vi "svx_Oct_Autoscale Ranges.vi"(10 "Display State In":T1={"X Scale Width %"=50.0, "Y Scale Height %"=50.0, "X-Axis Range"={"Minimum"=0.0, "Maximum"=10.0}, "Y-Axis Range"={"Minimum"=0.0, "Maximum"=10.0}, "Z-Axis Range"={"Minimum"=0.0, "Maximum"=10.0}, "Plot Color"=0, "Frame Color"=61212, "Background Color"=16252785, "Initial AutoScale Y"=TRUE, "AutoScale X"=2, "AutoScale Y"=2, "AutoScale Z"=2, "Plot Transparency"=FALSE, "X-Axis Name"="Frequency", "Y-Axis Name"="Amplitude", "Z-Axis Name"="", "X-Axis Scaling Factor"={"Offset"=0.0, "Multiplier"=1.0}, "Y-Axis Scaling Factor"={"Offset"=0.0, "Multiplier"=1.0}, "Z-Axis Scaling Factor"={"Offset"=0.0, "Multiplier"=1.0}, "X-Scale Visible"=TRUE, "Y-Scale Visible"=TRUE, "Z-Scale Visible"=TRUE, "X-Scale Label Visible"=TRUE, "Y-Scale Label Visible"=TRUE, "Z-Scale Label Visible"=TRUE, "X-Axis Range Scaled"={"Minimum"=0.0, "Maximum"=10.0}, "Y-Axis Range Scaled"={"Minimum"=0.0, "Maximum"=10.0}, "Z-Axis Range Scaled"={"Minimum"=0.0, "Maximum"=10.0}, "Rev Z Order"=FALSE, "X-Scale Format Str"="%#.4g", "Y-Scale Format Str"="%#.4g", "Z-Scale Format Str"="%#.4g", "Decor color"=12369084, "Scale Range Change"=refnum, "out of state queue"=refnum, "property nodes"=refnum} caption="State", 11 "Data Array In":T2={"z0"=0.0, "dz"=1.0, "Plots"=[]} {"Plots"."Y" format="%.2f"; "Plots"."X" format="%.2f"}) -> (0 "Cropped Info out":cluster{"First Index":i32, "Length":i32}, 1 "Update Ranges":bool[](array[boolean]), 2 "Display State Out":T1={"X Scale Width %"=50.0, "Y Scale Height %"=50.0, "X-Axis Range"={"Minimum"=0.0, "Maximum"=10.0}, "Y-Axis Range"={"Minimum"=0.0, "Maximum"=10.0}, "Z-Axis Range"={"Minimum"=0.0, "Maximum"=10.0}, "Plot Color"=0, "Frame Color"=61212, "Background Color"=16252785, "Initial AutoScale Y"=TRUE, "AutoScale X"=2, "AutoScale Y"=2, "AutoScale Z"=2, "Plot Transparency"=FALSE, "X-Axis Name"="Frequency", "Y-Axis Name"="Amplitude", "Z-Axis Name"="", "X-Axis Scaling Factor"={"Offset"=0.0, "Multiplier"=1.0}, "Y-Axis Scaling Factor"={"Offset"=0.0, "Multiplier"=1.0}, "Z-Axis Scaling Factor"={"Offset"=0.0, "Multiplier"=1.0}, "X-Scale Visible"=TRUE, "Y-Scale Visible"=TRUE, "Z-Scale Visible"=TRUE, "X-Scale Label Visible"=TRUE, "Y-Scale Label Visible"=TRUE, "Z-Scale Label Visible"=TRUE, "X-Axis Range Scaled"={"Minimum"=0.0, "Maximum"=10.0}, "Y-Axis Range Scaled"={"Minimum"=0.0, "Maximum"=10.0}, "Z-Axis Range Scaled"={"Minimum"=0.0, "Maximum"=10.0}, "Rev Z Order"=FALSE, "X-Scale Format Str"="%#.4g", "Y-Scale Format Str"="%#.4g", "Z-Scale Format Str"="%#.4g", "Decor color"=12369084, "Scale Range Change"=refnum, "out of state queue"=refnum, "property nodes"=refnum} caption="State", 3 "Data Array Out":T2={"z0"=0.0, "dz"=1.0, "Plots"=[]} {"Plots"."Y" format="%.2f"; "Plots"."X" format="%.2f"}, 4 "Update Autoscale":bool)   [LabVIEW 2017, in "SVX Octave Waterfall Graph.xctl"]
uses:
  <vilib>/addons/_XControls/Octave Waterfall Graph/SVX Octave Waterfall Graph.xctl
  <vilib>/addons/_XControls/Octave Waterfall Graph/subVIs/svx_Oct_Waterfall Data.ctl
  <vilib>/addons/_XControls/Octave Waterfall Graph/subVIs/svx_Oct_Waterfall State.ctl
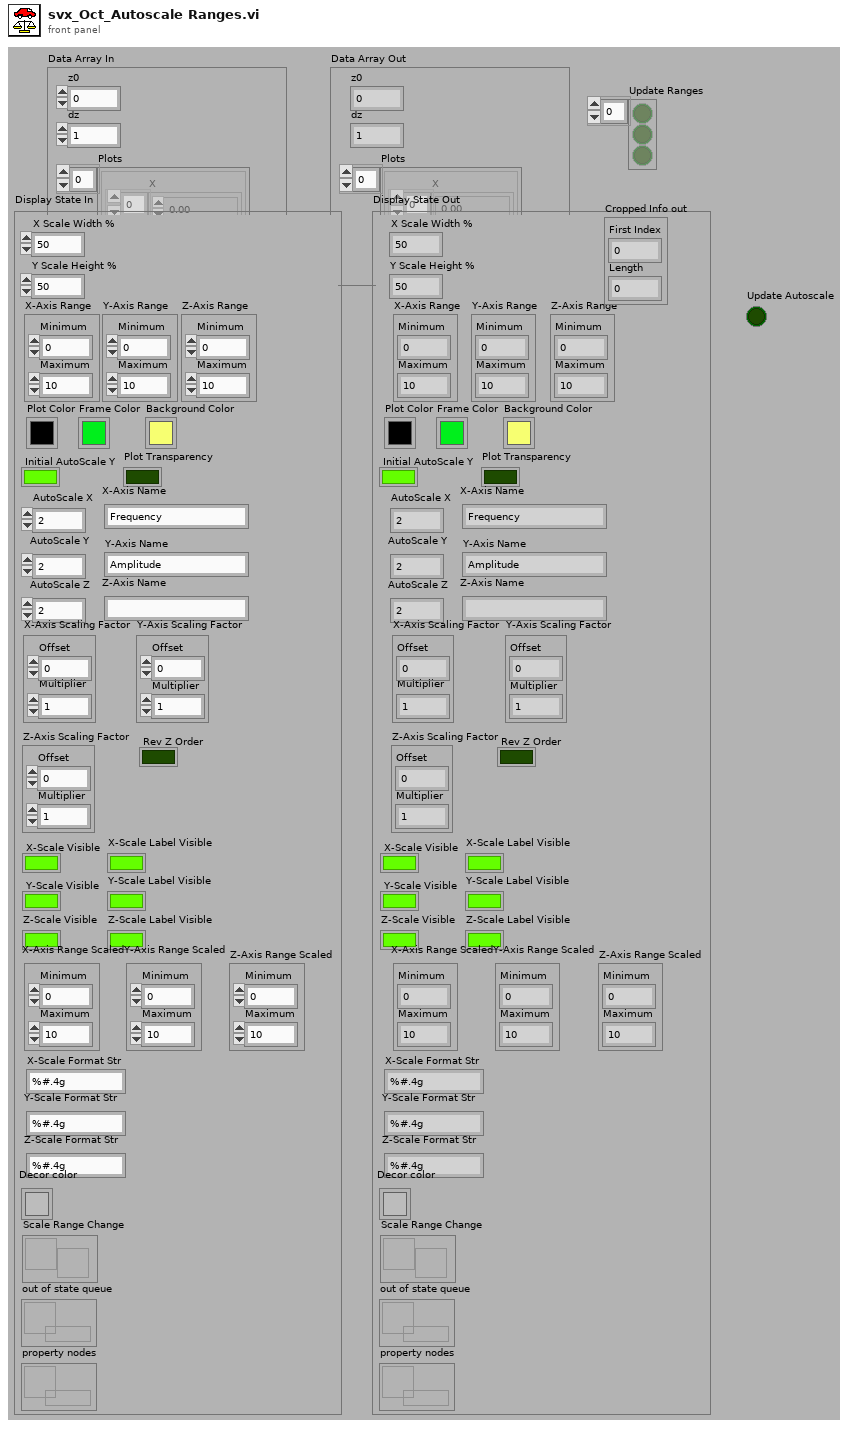
[diagram p1: front panel]
types:
  T1 = typedef "SVX Octave Waterfall Graph.xctl/svx_Oct_Waterfall State.ctl" = cluster{"X Scale Width %":dbl, "Y Scale Height %":dbl, "X-Axis Range":cluster{"Minimum":dbl, "Maximum":dbl}, "Y-Axis Range":cluster{"Minimum":dbl, "Maximum":dbl}, "Z-Axis Range":cluster{"Minimum":dbl, "Maximum":dbl}, "Plot Color":u32, "Frame Color":u32, "Background Color":u32, "Initial AutoScale Y":bool, "AutoScale X":u8, "AutoScale Y":u8, "AutoScale Z":u8, "Plot Transparency":bool, "X-Axis Name":string, "Y-Axis Name":string, "Z-Axis Name":string, "X-Axis Scaling Factor":cluster{"Offset":dbl, "Multiplier":dbl}, "Y-Axis Scaling Factor":cluster{"Offset":dbl, "Multiplier":dbl}, "Z-Axis Scaling Factor":cluster{"Offset":dbl, "Multiplier":dbl}, "X-Scale Visible":bool, "Y-Scale Visible":bool, "Z-Scale Visible":bool, "X-Scale Label Visible":bool, "Y-Scale Label Visible":bool, "Z-Scale Label Visible":bool, "X-Axis Range Scaled":cluster{"Minimum":dbl, "Maximum":dbl}, "Y-Axis Range Scaled":cluster{"Minimum":dbl, "Maximum":dbl}, "Z-Axis Range Scaled":cluster{"Minimum":dbl, "Maximum":dbl}, "Rev Z Order":bool, "X-Scale Format Str":string, "Y-Scale Format Str":string, "Z-Scale Format Str":string, "Decor color":u32, "Scale Range Change":refnum<user-event>, "out of state queue":refnum<queue>, "property nodes":refnum<queue>}
  T2 = typedef "SVX Octave Waterfall Graph.xctl/svx_Oct_Waterfall Data.ctl" = cluster{"z0":dbl, "dz":dbl, "Plots":cluster{"X":dbl[], "Y":dbl[]}[]}
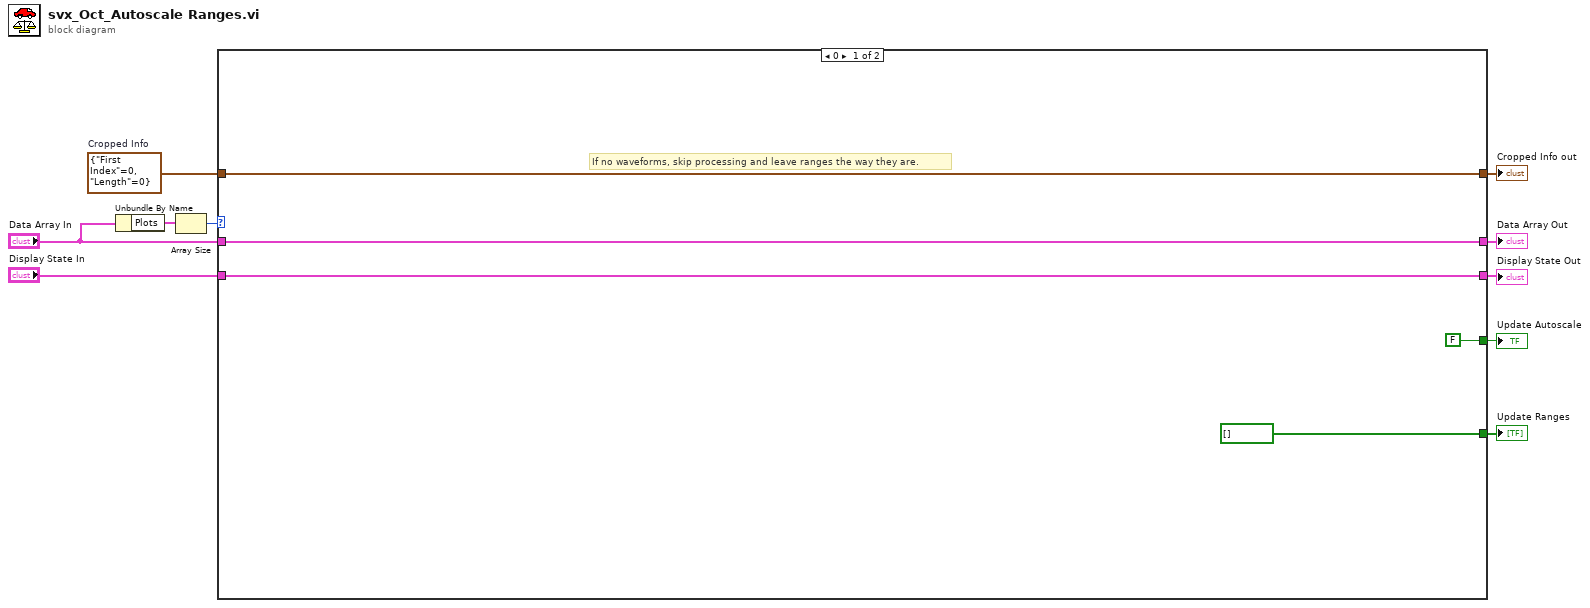
[diagram p0: block diagram]
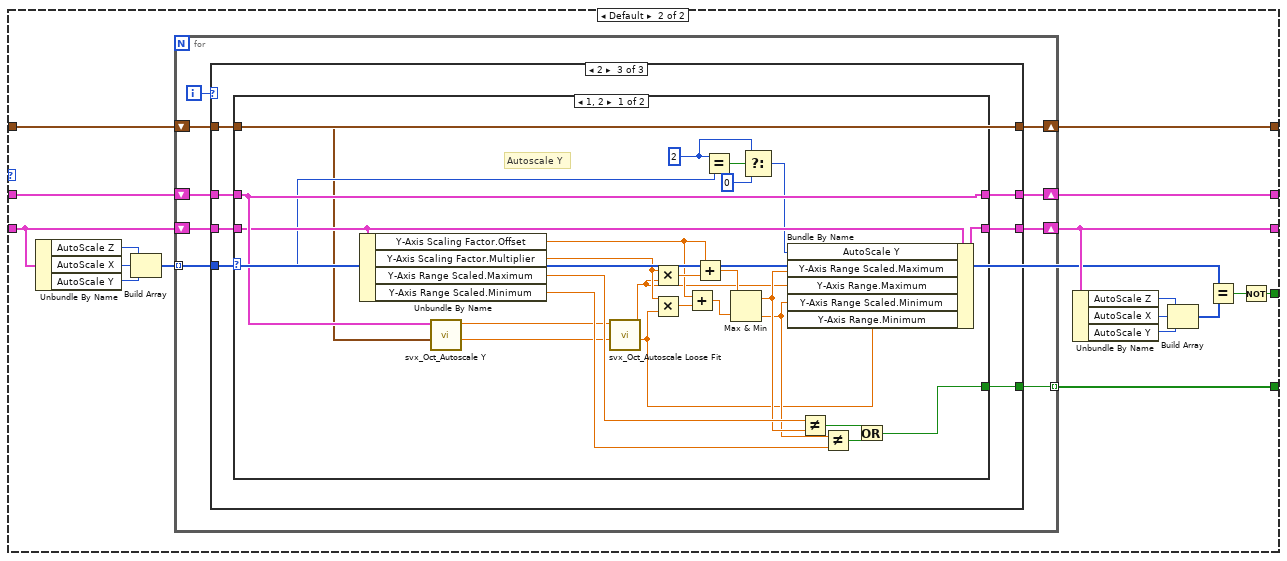
[diagram p2: hidden frame]
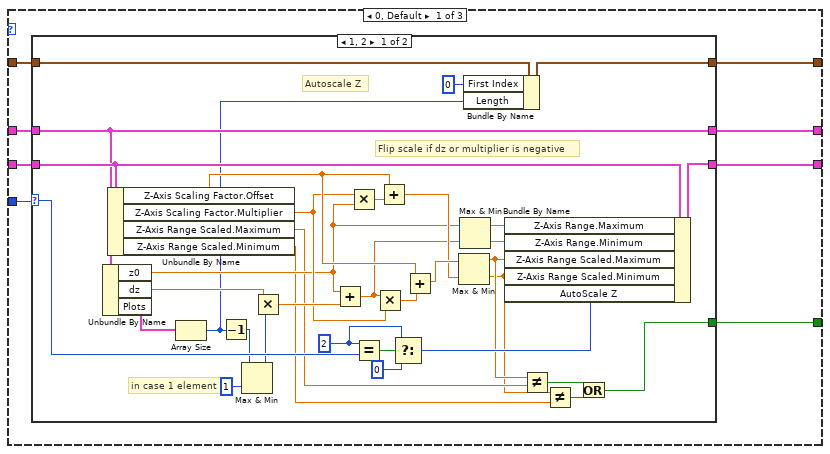
[diagram p3: hidden frame]
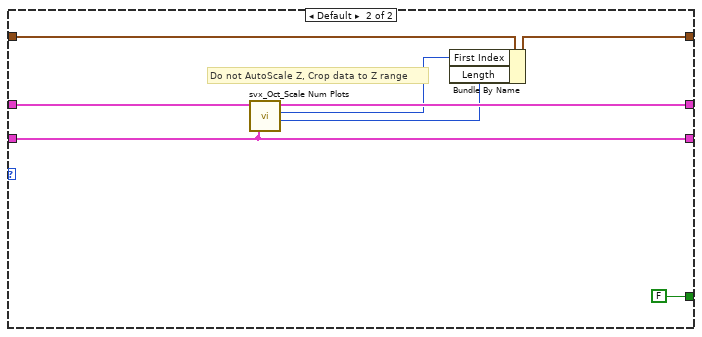
[diagram p4: hidden frame]
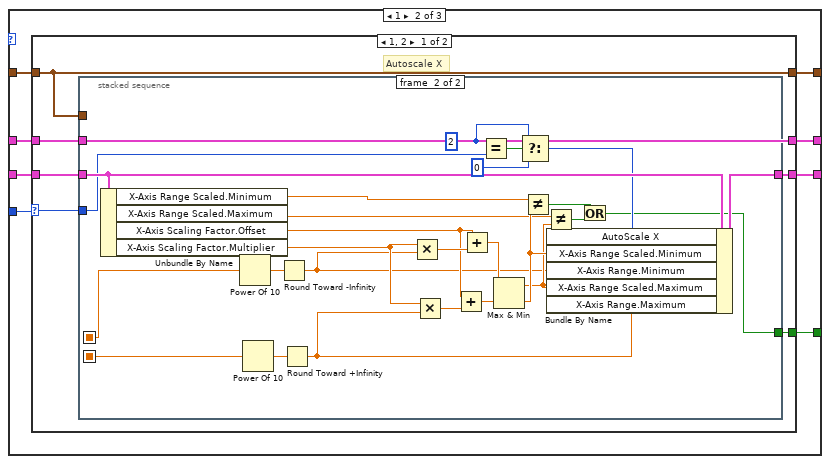
[diagram p5: hidden frame]
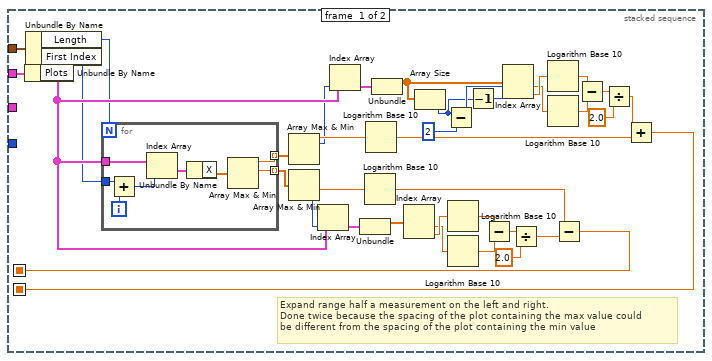
[diagram p6: hidden frame]
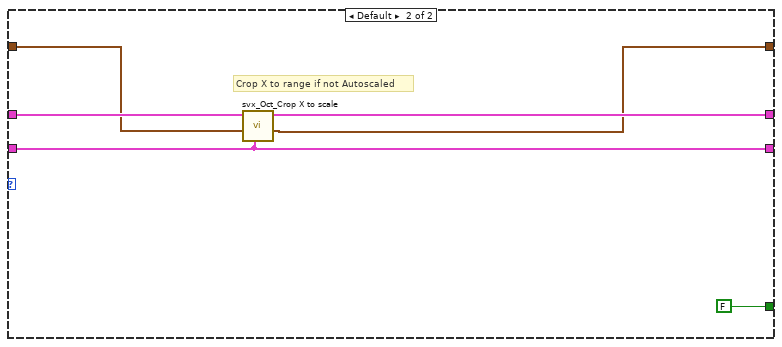
[diagram p7: hidden frame]
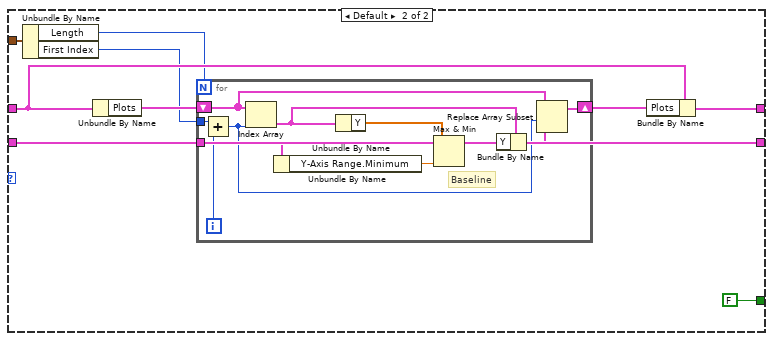
[diagram p8: hidden frame]
diagram:
  w3 = cluster{"First Index":i32, "Length":i32} {"First Index"=0, "Length"=0}  # Cropped Info
  n1 = Unbundle By Name("Data Array In") -> ("Plots"=w5:cluster{"X":dbl[], "Y":dbl[]}[])
  n2 = Array Size(array=w5) -> (size(s)=w7:i32)
  n3 = case shown="0" w7 {
    tunnel: [w14 w18] -> w10
    tunnel: "Display State In" -> [w14 w32]
    tunnel: "Data Array In" -> [w15 w28]
    tunnel: [w15 w27] -> w8
    tunnel: [bool[] [] w26] -> w4
    tunnel: w3 -> [w12 w25]
    tunnel: [w12 w24] -> w2
    tunnel: [FALSE w16] -> w1
    frame 0 {
      # "If no waveforms, skip processing and leave ranges the way they are."
    }
    frame Default {
      n4 = Unbundle By Name(w32) -> ("AutoScale Z"=w31:u8, "AutoScale X"=w30:u8, "AutoScale Y"=w29:u8)
      n5 = Build Array(w31, w30, w29) -> (w17:u8[])
      n6 = for {
        shift-right: [w40] -> w18
        shift-left: w32 -> [w41]
        tunnel: w17 -> [w37] mode=indexing
        shift-right: [w36] -> w27
        shift-left: w28 -> [w39]
        tunnel: [w35] -> w26 mode=indexing
        shift-right: [w33] -> w24
        shift-left: w25 -> [w34]
        i -> [w38]
        n7 = case shown="2" w38 {
          tunnel: w41 -> [w49 w100 w190]
          tunnel: [w48 w99 w189] -> w40
          tunnel: w39 -> [w47 w98 w188]
          tunnel: w37 -> [w46 w97 w187]
          tunnel: [w45 w96 w186] -> w36
          tunnel: [w44 w95 w185] -> w35
          tunnel: w34 -> [w43 w94 w184]
          tunnel: [w42 w93 w184] -> w33
          frame 0, Default {
            n8 = case shown="1, 2" w46 {
              selector: w46 -> [w65 _]
              tunnel: w49 -> [w83 w90]
              tunnel: [w84 w90] -> w48
              tunnel: w47 -> [w75 w92]
              tunnel: [w75 w91] -> w45
              tunnel: [w57 FALSE] -> w44
              tunnel: w43 -> [w55 w86]
              tunnel: [w54 w85] -> w42
              frame 1, 2 {
                w67 = u8 2 ("AutoScale Y")
                # "in case 1 element"
                # "Flip scale if dz or multiplier is negative"
                # "Autoscale Z"
                n9 = Unbundle By Name(w75) -> ("z0"=w71:dbl, "dz"=w77:dbl, "Plots"=w76:cluster{"X":dbl[], "Y":dbl[]}[])
                n10 = Unbundle By Name(w83) -> ("Z-Axis Scaling Factor.Offset"=w80:dbl, "Z-Axis Scaling Factor.Multiplier"=w78:dbl, "Z-Axis Range Scaled.Maximum"=w61:dbl, "Z-Axis Range Scaled.Minimum"=w59:dbl)
                n11 = Array Size(array=w76) -> (size(s)=w53:i32)
                n12 = Decrement(x=w53) -> (x-1=w51:i32)
                n13 = Max & Min(x=w51, y=1) -> (max(x,y)=w50:i32)  [unwired: 1 out]
                n14 = Multiply(x=w77, y=w50) -> (x*y=w79:dbl)
                n15 = Add(x=w71, y=w79) -> (x+y=w72:dbl)
                n16 = Multiply(x=w78, y=w71) -> (x*y=w82:dbl)
                n17 = Equal?(x=w67, y=w65) -> (x = y?=w68:bool)
                n18 = Multiply(x=w72, y=w78) -> (x*y=w81:dbl)
                n19 = Add(x=w80, y=w82) -> (x+y=w73:dbl)
                n20 = Select(t=w67, s=w68, f=u8 0 ("AutoScale Y")) -> (s? t:f=w64:u8)
                n21 = Add(x=w80, y=w81) -> (x+y=w74:dbl)
                n22 = Max & Min(x=w74, y=w73) -> (max(x,y)=w60:dbl, min(x,y)=w58:dbl)
                n23 = Max & Min(x=w71, y=w72) -> (max(x,y)=w70:dbl, min(x,y)=w69:dbl)
                n24 = Bundle By Name(cluster=w55, "First Index"=0, "Length"=w53) -> (w54:cluster{"First Index":i32, "Length":i32})
                n25 = Bundle By Name(cluster=w83, "Z-Axis Range.Maximum"=w70, "Z-Axis Range.Minimum"=w69, "Z-Axis Range Scaled.Maximum"=w60, "Z-Axis Range Scaled.Minimum"=w58, "AutoScale Z"=w64) -> (w84:T1)
                n26 = Not Equal?(x=w60, y=w61) -> (x != y?=w63:bool)
                n27 = Not Equal?(x=w58, y=w59) -> (x != y?=w62:bool)
                n28 = Or(x=w63, y=w62) -> (x .or. y?=w57:bool)
              }
              frame Default {
                # "Do not AutoScale Z, Crop data to Z range"
                n29 = call <vilib>:"svx_Oct_Scale Num Plots.vi"("Display State In"=w90, "Waveform Array In"=w92) -> ("Z length"=w87:i32, "Z Index"=w88:i32, "Waveform Array Out"=w91:T2)  [unwired: 7 in]
                n30 = Bundle By Name(cluster=w86, "First Index"=w88, "Length"=w87) -> (w85:cluster{"First Index":i32, "Length":i32})
              }
            }
          }
          frame 1 {
            n31 = case shown="1, 2" w97 {
              selector: w97 -> [w104 _]
              tunnel: w100 -> [w105 w182]
              tunnel: [w103 w182] -> w99
              tunnel: w98 -> [w106 w183]
              tunnel: [w106 w181] -> w96
              tunnel: [w102 FALSE ("Boolean")] -> w95
              tunnel: w94 -> [w101 w178]
              tunnel: [w101 w179] -> w93
              frame 1, 2 {
                # "Autoscale X"
                n32 = stacked-sequence {
                  seq-local: [w110 _] -> [_ w157]
                  seq-local: [w111 _] -> [_ w155]
                  tunnel: w106 -> [w143 _]
                  tunnel: w105 -> [_ w177]
                  tunnel: w104 -> [_ w160]
                  tunnel: [_ w159] -> w103
                  tunnel: [_ w158] -> w102
                  tunnel: w101 -> [w109 _]
                  frame #0 {
                    # "Expand range half a measurement on the left and right. \nDone twice because the spacing of the plot containing the max value could\nbe different from the spacing of the plot containing the min value"
                    n33 = Unbundle By Name(w143) -> ("Plots"=w123:cluster{"X":dbl[], "Y":dbl[]}[])
                    n34 = Unbundle By Name(w109) -> ("Length"=w108:i32, "First Index"=w107:i32)
                    n35 = for {
                      N: w108 -> [_]
                      tunnel: w123 -> [w148]
                      tunnel: [w150] -> w142 mode=indexing
                      tunnel: [w149] -> w141 mode=indexing
                      tunnel: w107 -> [w144]
                      i -> [w146]
                      n36 = Add(x=w144, y=w146) -> (x+y=w145:i32)
                      n37 = Index Array(array=w148, index=w145) -> (element=w147:cluster{"X":dbl[], "Y":dbl[]})
                      n38 = Unbundle By Name(w147) -> ("X"=w151:dbl[])
                      n39 = Array Max & Min(array=w151) -> (max value=w150:dbl, min value=w149:dbl)  [unwired: 2 out]
                    }
                    n40 = Array Max & Min(array=w142) -> (max value=w132:dbl, max index (indices)=w122:i32)  [unwired: 2 out]
                    n41 = Array Max & Min(array=w141) -> (min value=w130:dbl, min index (indices)=w140:i32)  [unwired: 2 out]
                    n42 = Index Array(array=w123, index=w140) -> (element=w139:cluster{"X":dbl[], "Y":dbl[]})
                    n43 = Index Array(array=w123, index=w122) -> (element=w124:cluster{"X":dbl[], "Y":dbl[]})
                    n44 = Unbundle(w139) -> ("X"=w136:dbl[])  [unwired: 1 out]
                    n45 = Logarithm Base 10(1:w130) -> (0:w129:dbl)
                    n46 = Logarithm Base 10(1:w132) -> (0:w131:dbl)
                    n47 = Unbundle(w124) -> ("X"=w120:dbl[])  [unwired: 1 out]
                    n48 = Index Array(array=w136) -> (element #1=w114:dbl, element #2=w115:dbl)  [unwired: 2 in]
                    n49 = Array Size(array=w120) -> (size(s)=w116:i32)
                    n50 = Subtract(x=w116, y=2) -> (x-y=w118:i32)
                    n51 = Logarithm Base 10(1:w115) -> (0:w134:dbl)
                    n52 = Logarithm Base 10(1:w114) -> (0:w135:dbl)
                    n53 = Decrement(x=w116) -> (x-1=w117:i32)
                    n54 = Subtract(x=w134, y=w135) -> (x-y=w137:dbl)
                    n55 = Index Array(array=w120, index #1=w118, index #2=w117) -> (element #1=w112:dbl, element #2=w113:dbl)
                    n56 = Divide(x=w137, y=2.0) -> (x/y=w133:dbl)
                    n57 = Logarithm Base 10(1:w113) -> (0:w128:dbl)
                    n58 = Logarithm Base 10(1:w112) -> (0:w127:dbl)
                    n59 = Subtract(x=w129, y=w133) -> (x-y=w110:dbl)
                    n60 = Subtract(x=w128, y=w127) -> (x-y=w126:dbl)
                    n61 = Divide(x=w126, y=2.0) -> (x/y=w121:dbl)
                    n62 = Add(x=w121, y=w131) -> (x+y=w111:dbl)
                  }
                  frame #1 {
                    w169 = u8 2 ("AutoScale Y")
                    n63 = Unbundle By Name(w177) -> ("X-Axis Range Scaled.Minimum"=w161:dbl, "X-Axis Range Scaled.Maximum"=w165:dbl, "X-Axis Scaling Factor.Offset"=w173:dbl, "X-Axis Scaling Factor.Multiplier"=w174:dbl)
                    n64 = Power Of 10(x=w157) -> (10^x=w156:dbl)
                    n65 = Power Of 10(x=w155) -> (10^x=w154:dbl)
                    n66 = Round Toward -Infinity(1:w156) -> (0:w153:dbl)
                    n67 = Round Toward +Infinity(x=w154) -> (ceil(x): smallest int >= x=w152:dbl)
                    n68 = Multiply(x=w174, y=w153) -> (x*y=w176:dbl)
                    n69 = Multiply(x=w174, y=w152) -> (x*y=w175:dbl)
                    n70 = Add(x=w173, y=w175) -> (x+y=w172:dbl)
                    n71 = Add(x=w173, y=w176) -> (x+y=w171:dbl)
                    n72 = Equal?(x=w169, y=w160) -> (x = y?=w170:bool)
                    n73 = Max & Min(x=w171, y=w172) -> (max(x,y)=w164:dbl, min(x,y)=w166:dbl)
                    n74 = Select(t=w169, s=w170, f=u8 0 ("AutoScale Y")) -> (s? t:f=w167:u8)
                    n75 = Not Equal?(x=w161, y=w166) -> (x != y?=w163:bool)
                    n76 = Not Equal?(x=w165, y=w164) -> (x != y?=w162:bool)
                    n77 = Bundle By Name(cluster=w177, "AutoScale X"=w167, "X-Axis Range Scaled.Minimum"=w166, "X-Axis Range.Minimum"=w153, "X-Axis Range Scaled.Maximum"=w164, "X-Axis Range.Maximum"=w152) -> (w159:T1)
                    n78 = Or(x=w163, y=w162) -> (x .or. y?=w158:bool)
                  }
                }
              }
              frame Default {
                # "Crop X to range if not Autoscaled"
                n79 = call <vilib>:"svx_Oct_Crop X to scale.vi"("Display State In"=w182, "Cropped Info"=w178, "Waveform Array In"=w183) -> ("Cropped Info out"=w179:cluster{"First Index":i32, "Length":i32}, "Waveform Array Out"=w181:T2)  [unwired: 7 in]
              }
            }
          }
          frame 2 {
            n80 = case shown="1, 2" w187 {
              selector: w187 -> [w207 _]
              tunnel: w190 -> [w214 w225]
              tunnel: [w216 w225] -> w189
              tunnel: w188 -> [w215 w224]
              tunnel: [w215 w223] -> w186
              tunnel: [w196 FALSE] -> w185
              tunnel: w184 -> [w195 w221]
              frame 1, 2 {
                w205 = u8 2 ("AutoScale Y")
                # "Autoscale Y"
                n81 = Unbundle By Name(w214) -> ("Y-Axis Scaling Factor.Offset"=w210:dbl, "Y-Axis Scaling Factor.Multiplier"=w211:dbl, "Y-Axis Range Scaled.Maximum"=w200:dbl, "Y-Axis Range Scaled.Minimum"=w198:dbl)
                n82 = call <vilib>:"svx_Oct_Autoscale Y.vi"("Cropped Info"=w195, "Data Array In"=w215) -> ("min"=w194:dbl, "max"=w193:dbl)  [unwired: 8 in]
                n83 = call <vilib>:"svx_Oct_Autoscale Loose Fit.vi"("Min"=w194, "Max"=w193) -> ("Loose Fit Min"=w191:dbl, "Loose Fit Max"=w192:dbl)  [unwired: 8 in]
                n84 = Multiply(x=w211, y=w192) -> (x*y=w213:dbl)
                n85 = Multiply(x=w211, y=w191) -> (x*y=w212:dbl)
                n86 = Add(x=w210, y=w212) -> (x+y=w209:dbl)
                n87 = Add(x=w210, y=w213) -> (x+y=w208:dbl)
                n88 = Equal?(x=w205, y=w207) -> (x = y?=w206:bool)
                n89 = Max & Min(x=w208, y=w209) -> (max(x,y)=w199:dbl, min(x,y)=w197:dbl)
                n90 = Select(t=w205, s=w206, f=u8 0 ("AutoScale Y")) -> (s? t:f=w203:u8)
                n91 = Bundle By Name(cluster=w214, "AutoScale Y"=w203, "Y-Axis Range Scaled.Maximum"=w199, "Y-Axis Range.Maximum"=w192, "Y-Axis Range Scaled.Minimum"=w197, "Y-Axis Range.Minimum"=w191) -> (w216:T1)
                n92 = Not Equal?(x=w200, y=w199) -> (x != y?=w202:bool)
                n93 = Not Equal?(x=w197, y=w198) -> (x != y?=w201:bool)
                n94 = Or(x=w202, y=w201) -> (x .or. y?=w196:bool)
              }
              frame Default {
                n95 = Unbundle By Name(w221) -> ("Length"=w220:i32, "First Index"=w218:i32)
                n96 = Unbundle By Name(w224) -> ("Plots"=w219:cluster{"X":dbl[], "Y":dbl[]}[])
                n97 = for {
                  N: w220 -> [_]
                  tunnel: w225 -> [w236]
                  shift-right: [w229] -> w217
                  shift-left: w219 -> [w228]
                  tunnel: w218 -> [w231]
                  i -> [w232]
                  # "Baseline"
                  n98 = Add(x=w231, y=w232) -> (x+y=w226:i32)
                  n99 = Index Array(array=w228, index=w226) -> (element=w230:cluster{"X":dbl[], "Y":dbl[]})
                  n100 = Unbundle By Name(w236) -> ("Y-Axis Range.Minimum"=w234:dbl)
                  n101 = Unbundle By Name(w230) -> ("Y"=w235:dbl[])
                  n102 = Max & Min(x=w235, y=w234) -> (max(x,y)=w233:dbl[])  [unwired: 1 out]
                  n103 = Bundle By Name(cluster=w230, "Y"=w233) -> (w227:cluster{"X":dbl[], "Y":dbl[]})
                  n104 = Replace Array Subset(array=w228, new element=w227, index=w226) -> (w229:cluster{"X":dbl[], "Y":dbl[]}[])
                }
                n105 = Bundle By Name(cluster=w224, "Plots"=w217) -> (w223:T2)
              }
            }
          }
        }
      }
      n106 = Unbundle By Name(w18) -> ("AutoScale Z"=w20:u8, "AutoScale X"=w21:u8, "AutoScale Y"=w22:u8)
      n107 = Build Array(w20, w21, w22) -> (w19:u8[])
      n108 = Equal?(x=w17, y=w19) -> (x = y?=w23:bool)
      n109 = Not(x=w23) -> (.not. x?=w16:bool)
    }
  }
  "Data Array Out" <- w8
  "Display State Out" <- w10
  "Update Ranges" <- w4
  "Cropped Info out" <- w2
  "Update Autoscale" <- w1
